vi "TransferItems.vi"(8 "error in (no error)":errorcluster, 10 "Session":refnum<class "Session.lvclass">, 11 "TransferFolder in":refnum<class "TransferFolder-Get.lvclass">) -> (0 "error out":errorcluster, 3 "FileTransfer out":refnum<class "TransferFolder-Get.lvclass">)   [LabVIEW 2015, in "WinSCP.lvlib" / "TransferFolder-Get.lvclass"]
uses:
  TransferFolder-Get.lvclass
  Session/Session.lvclass
  C:/Users/Public/Documents/Projects/lv-winscp/Bin WinSCP/WinSCPnet.dll
  Bin WinSCP/WinSCPnet.dll
  FileTransferOptions/FileTransferOptions.lvclass
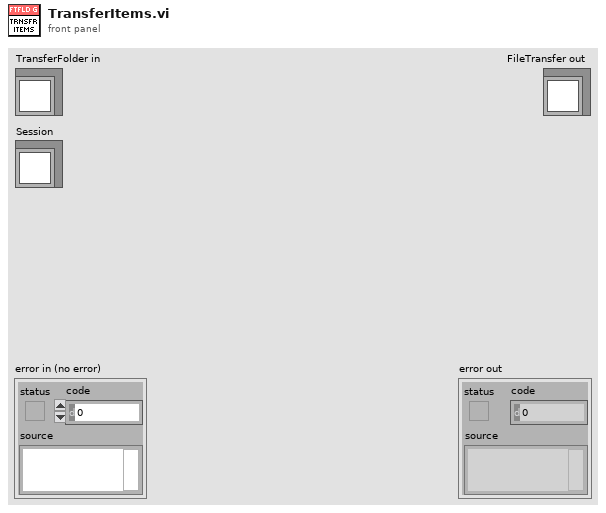
[diagram p1: front panel]
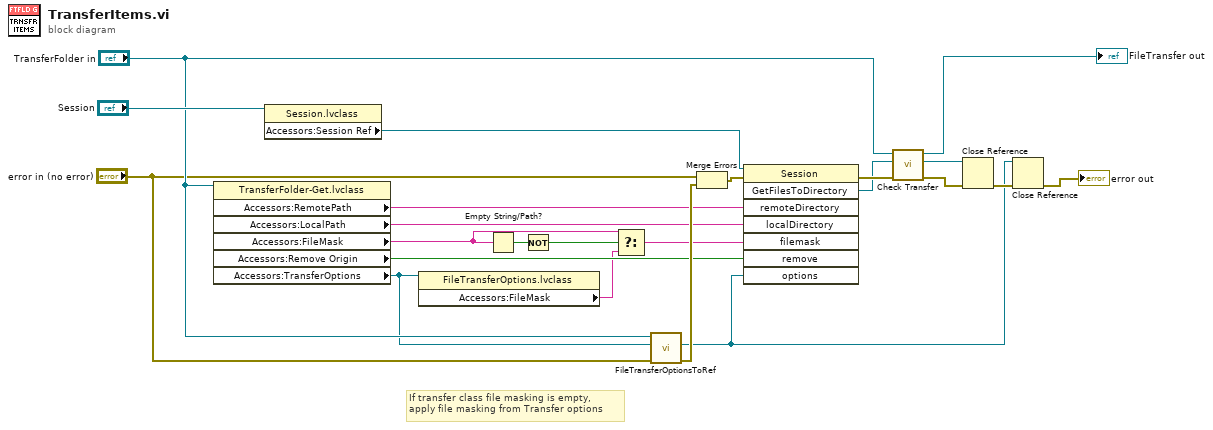
[diagram p0: block diagram]
diagram:
  # "If transfer class file masking is empty,\napply file masking from Transfer options"
  n1 = property class="TransferFolder-Get.lvclass"(reference="TransferFolder in") -> ("Accessors:RemotePath"=w22:string, "Accessors:LocalPath"=w21:string, "Accessors:FileMask"=w4:string, "Accessors:Remove Origin"=w20:bool, "Accessors:TransferOptions"=w6:refnum<class "FileTransferOptions.lvclass">)  [unwired: 1 in, 2 out]
  n2 = property class="Session.lvclass"(reference="Session") -> ("Accessors:Session Ref"=w16:refnum<k24>)  [unwired: 1 in, 2 out]
  n3 = property class="FileTransferOptions.lvclass"(reference=w6) -> ("Accessors:FileMask"=w2:string)  [unwired: 1 in, 2 out]
  n4 = Empty String/Path?(string/path=w4) -> (empty?=w5:bool)
  n5 = Not(x=w5) -> (.not. x?=w1:bool)
  n6 = Select(t=w4, s=w1, f=w2) -> (s? t:f=w3:string)
  n7 = call-dynamic "FileTransferOptionsToRef.vi"("error in (no error)"="error in (no error)", "FileTransferOptions"=w6, "FileTransfer in"="TransferFolder in") -> ("error out"=w23:errorcluster, "TransferOptions Ref"=w9:refnum<k24>)  [unwired: 7 in]
  n8 = Merge Errors("error in (no error)", w23) -> (w7:errorcluster)
  n9 = invoke class="Session" method="GetFilesToDirectory"(reference=w16, error in=w7, "remoteDirectory"=w22, "localDirectory"=w21, "filemask"=w3, "remove"=w20, "options"=w9) -> (error out=w19:errorcluster, "GetFilesToDirectory"=w18:refnum<k24>)  [unwired: 1 in, 6 out]
  n10 = call-dynamic "Check Transfer.vi"("error in"=w19, "TransferOperationResult in"=w18, "FileTransfer in"="TransferFolder in") -> ("error out"=w14:errorcluster, "TransferOperationResult out"=w15:refnum<k24>, "FileTransfer out"=→"FileTransfer out":refnum<class "TransferFolder-Get.lvclass">)  [unwired: 6 in]
  n11 = Close Reference(reference=w15, error in (no error)=w14) -> (error out=w11:errorcluster)
  n12 = Close Reference(reference=w9, error in (no error)=w11) -> (error out=→"error out":errorcluster)
